vi "Utility Reset USB Communication Config.vi"(7 "Retry Attempts (0)":i32 min=0, 8 "error in (no error)":errorcluster, 11 "VISA resource name (in)":refnum<visa-resource-name>) -> (0 "error out":errorcluster, 2 "Response Cluster":T1 {"Command ID" format="%x"}, 3 "VISA resource name (out)":refnum<visa-resource-name>)   [LabVIEW 2020, in "Omega Platinum Series.lvlib"]
doc: "Configures the USB Communication for the Omega Platinum Series temperature controller."
uses:
  <instrlib>/RxnRover/OmegaPlatinumSeriesDriver/Omega Platinum Series.lvlib
  <instrlib>/RxnRover/OmegaPlatinumSeriesDriver/Public/Type Defs/Response.ctl
panel:
  out "Command":string
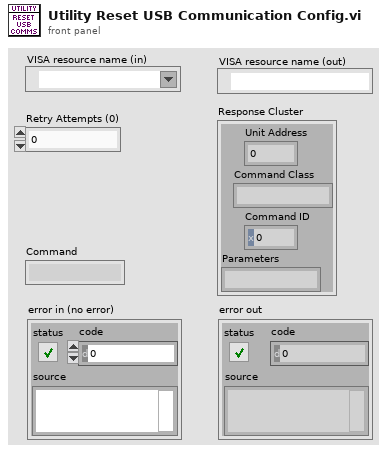
[diagram p1: front panel]
types:
  T1 = typedef "Omega Platinum Series.lvlib/Response.ctl" = cluster{"Unit Address":i32, "Command Class":string, "Command ID":u32, "Parameters":string}
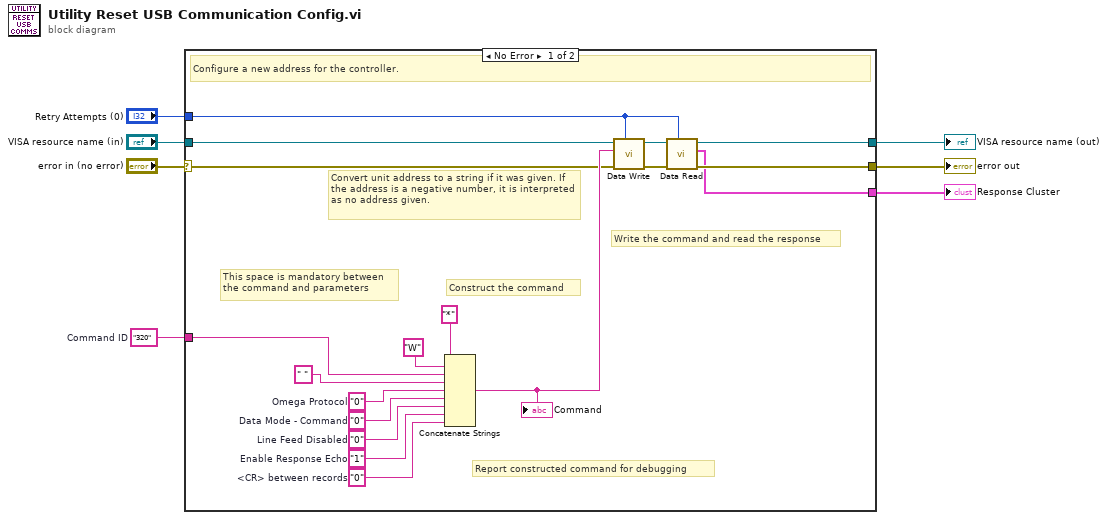
[diagram p0: block diagram]
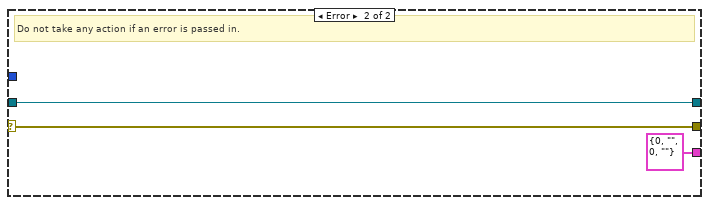
[diagram p2: hidden frame]
diagram:
  w7 = "320"  # Command ID
  n1 = case shown="No Error" "error in (no error)" {
    selector: "error in (no error)" -> [w23 w28]
    tunnel: w7 -> [w16 _]
    tunnel: [w19 w28] -> w5
    tunnel: "VISA resource name (in)" -> [w25 w27]
    tunnel: [w20 w27] -> w3
    tunnel: [w18 T1 {"Unit Address"=0, "Command Class"="", "Command ID"=0, "Parameters"=""} ("Response Cluster")] -> w2
    tunnel: "Retry Attempts (0)" -> [w8 _]
    frame No Error {
      w12 = "0"  # <CR> between records
      w11 = "1"  # Enable Response Echo
      w10 = "0"  # Line Feed Disabled
      w9 = "0"  # Data Mode - Command
      w13 = "0"  # Omega Protocol
      # "Report constructed command for debugging"
      # "Write the command and read the response"
      # "This space is mandatory between\nthe command and parameters"
      # "Convert unit address to a string if it was given. If the address is a negative number, it is interpreted as no address given."
      # "Construct the command"
      # "Configure a new address for the controller."
      n2 = Concatenate Strings("*" ("string"), "W" ("string"), w16, " " ("string"), w13, w9, w10, w11, w12) -> (w24:string)
      "Command" <- w24
      n3 = call <instrlib>:"Data Write.vi"("Retry Attempts (0)"=w8, "error in (no error)"=w23, "Command"=w24, "VISA Refnum in"=w25) -> ("error out"=w22:errorcluster, "VISA Refnum out"=w21:refnum<visa-resource-name>)  [unwired: 6 in]
      n4 = call <instrlib>:"Data Read.vi"("Retry Attempts (0)"=w8, "error in (no error)"=w22, "VISA Refnum in"=w21) -> ("error out"=w19:errorcluster, "Response Cluster"=w18:T1, "VISA Refnum out"=w20:refnum<visa-resource-name>)  [unwired: 5 in, 1 out]
    }
    frame Error {
      # "Do not take any action if an error is passed in."
    }
  }
  "error out" <- w5
  "VISA resource name (out)" <- w3
  "Response Cluster" <- w2
